vi "Main.vi"() -> (11 "server endpoint URL":string="opc.tcp://10.131.1.22:4840")   [LabVIEW 2018, in "OPC UA.lvlib"]
uses:
  OPC UA.lvlib
  support/Message Queue/Message Cluster.ctl
  <vilib>/Utility/miscctls.llb/LVPoint32TypeDef.ctl
  controls/UI State.ctl
  OPC Module Config.ctl
  Scale Module Folder/Measure Instrument/State Enum.ctl
  OPC Settings.ctl
  Variable Data Cluster.ctl
  <vilib>/OPCUA/controls/NodeId.ctl
  <vilib>/OPCUA/controls/OPC UA StatusCode.ctl
  <vilib>/OPCUA/controls/Subscription ID.ctl
  <vilib>/OPCUA/controls/OPC UA Client Refnum.ctl
  <vilib>/OPCUA/controls/Subscription Data Change.ctl
  <vilib>/OPCUA/controls/Data Type.ctl
  OPC Display Cluster.ctl
  support/Message Queue/Enqueue Message (Single).vi
  <vilib>/Utility/error.llb/Error Cluster From Error Code.vi
  <vilib>/ErrorRing/Error Ring.xnode
  support/Message Queue/Message Queue.lvlib
  support/Support Library.lvlib
  support/Command Log VIs/Command Logging.lvlib
  support/User Event - Stop/User Event - Stop.lvlib
  Scale Module Folder/Measure Instrument/Scale Module Engine.lvlib
  OPC Dialog.vi
panel:
  out "Updating":bool
  in  "Name of Parent Panel":string="Main.vi"
  in  "New Center Coords":T1={"Horizontal"=470, "Vertical"=200}
  in  "Config":variant
  in  "Main UI Message Queue":refnum<queue>
  out "ScanCode":i16
  in  "Settings Button":bool
  in  "Exit":bool
  out "Status":string
  out "Log File path":path
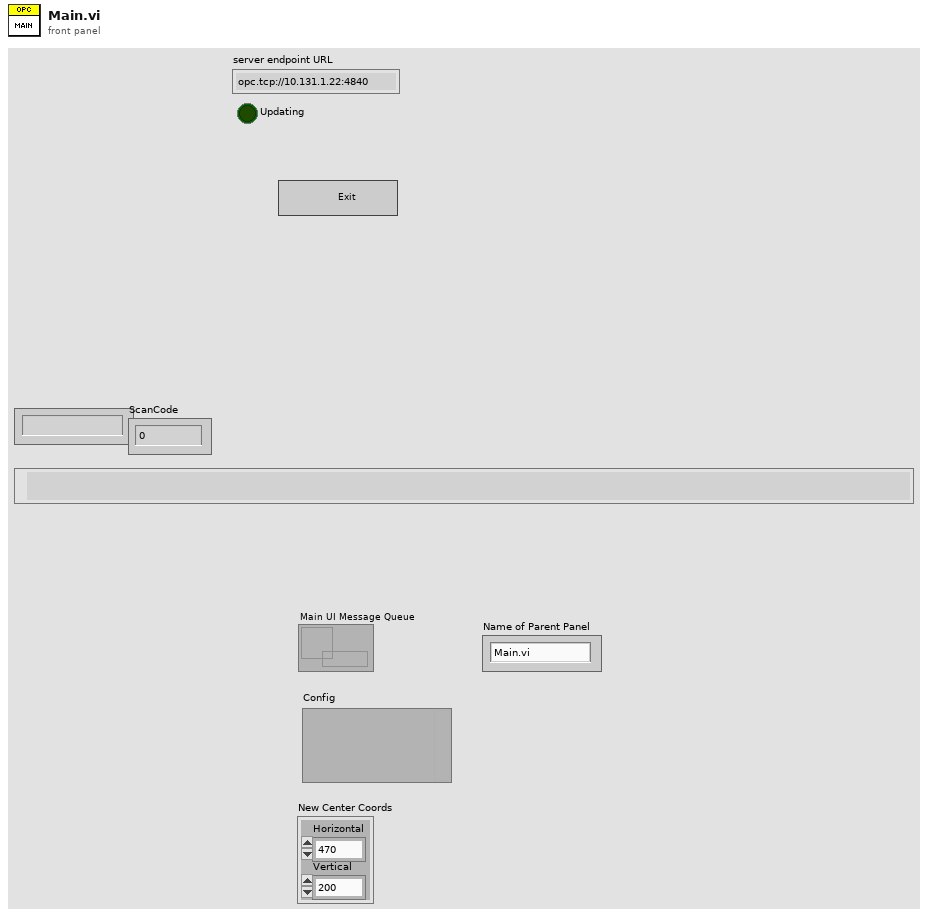
[diagram p1: front panel]
types:
  T1 = typedef "LVPoint32TypeDef.ctl" = cluster{"Horizontal":i32, "Vertical":i32}
  T2 = typedef "UI State.ctl" = enum16{"Idle", "Acquiring and Logging", "Waiting for Exit", "Waiting for Exit (Acq Stopped)", "Waiting for Exit (Log Stopped)", "Waiting for Stop", "Waiting for Stop (Acq Stopped)", "Waiting for Stop (Log Stopped)"}
  T3 = typedef "OPC UA.lvlib/OPC Module Config.ctl" = cluster{"State":T4, "GUID":string, "Drop Coords":T1, "Configuration":T5, "First Iteration":bool, "Data":cluster{"Object Name":string, "Variable Array":T6[]}[], "Process Name":string, "Load Count":i32, "Log Started":bool, "subscription ID out":T9, "OPC UA client refnum out":T10, "Event Registration Refnum":refnum<event-registration>, "Start Time":timestamp, "Current Time":timestamp}
  T4 = typedef "Scale Module.lvlib/Scale Module Engine.lvlib/State Enum.ctl" = enum16{"Measuring", "Idle"}
  T5 = typedef "OPC UA.lvlib/OPC Settings.ctl" = cluster{"Cycle Period":dbl, "server endpoint URL":string, "security policy":cluster{"message mode":enum16{"None", "Sign", "Sign and Encrypt"}, "security":enum16{"Basic256", "Basic128Rsa15"}}, "Trust Any Server":bool}
  T6 = typedef "OPC UA.lvlib/Variable Data Cluster.ctl" = cluster{"node ID":T7, "browse name":string, "status":T8, "timestamp":timestamp, "value ":variant}
  T7 = typedef "NodeId.ctl" = string
  T8 = typedef "OPC UA StatusCode.ctl" = u32
  T9 = typedef "Subscription ID.ctl" = u32
  T10 = typedef "OPC UA Client Refnum.ctl" = refnum<k21>
  T11 = typedef "OPC UA.lvlib/Message Queues.ctl" = cluster{"OPC UI":refnum<queue>, "OPC Engine":refnum<queue>, "OPC Display":refnum<queue>}
  T12 = typedef "OPC UA.lvlib/OPC Display Cluster.ctl" = cluster{"URL":string, "Cycle":i32, "Updating":bool}
  T13 = cluster{"Shift":bool, "Ctrl":bool, "Alt":bool, "Cmd":bool, "Opt":bool}
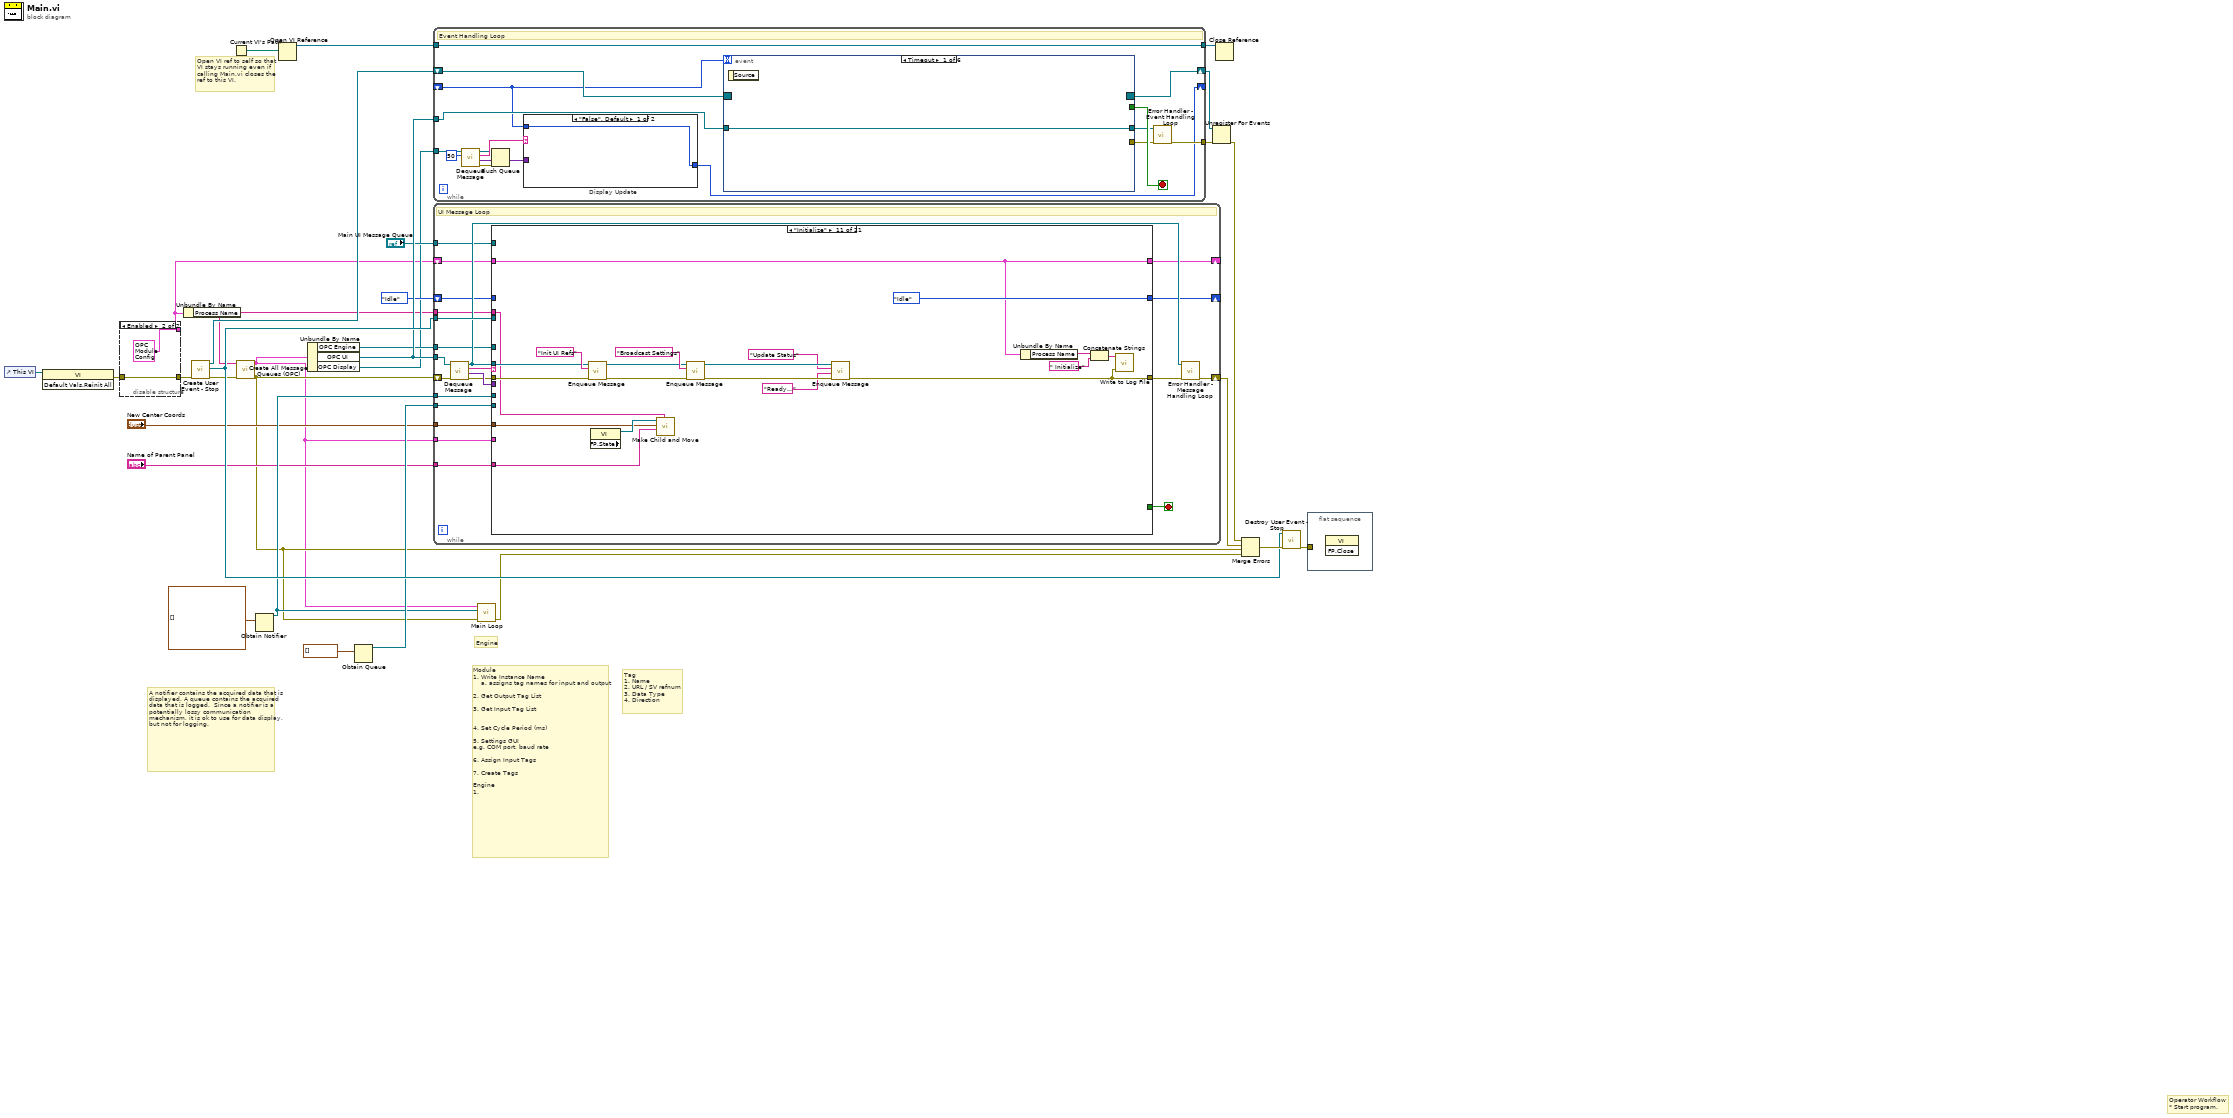
[diagram p0: block diagram]
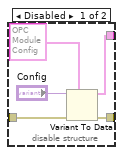
[diagram p2: hidden frame]
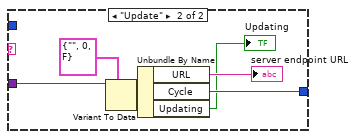
[diagram p3: hidden frame]
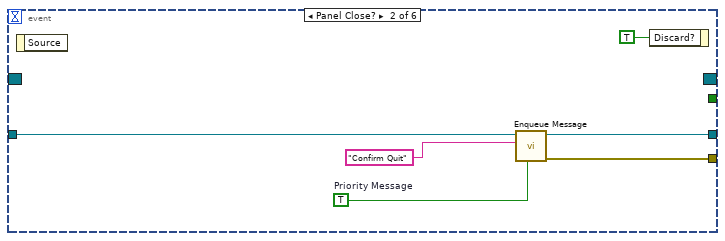
[diagram p4: hidden frame]
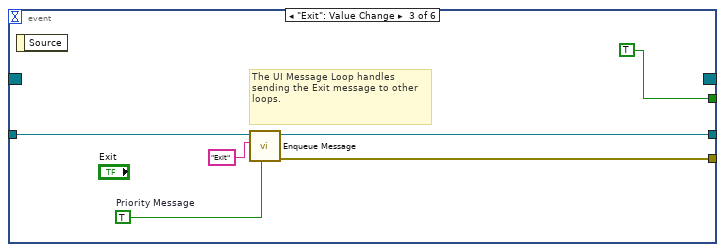
[diagram p5: hidden frame]
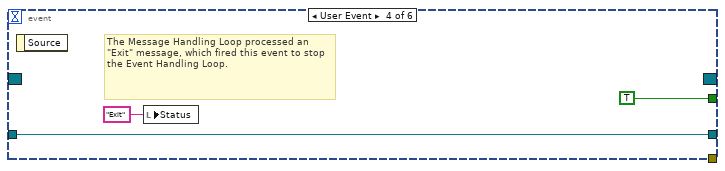
[diagram p6: hidden frame]
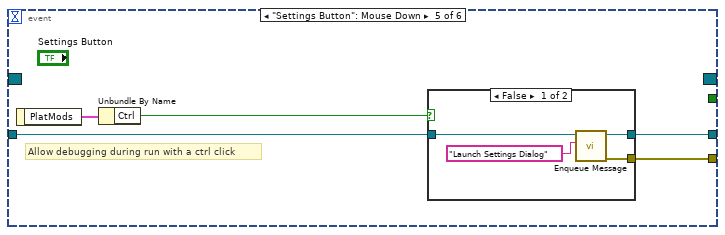
[diagram p7: hidden frame]
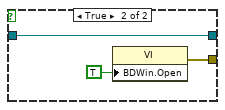
[diagram p8: hidden frame]
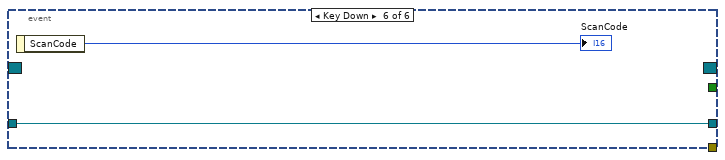
[diagram p9: hidden frame]
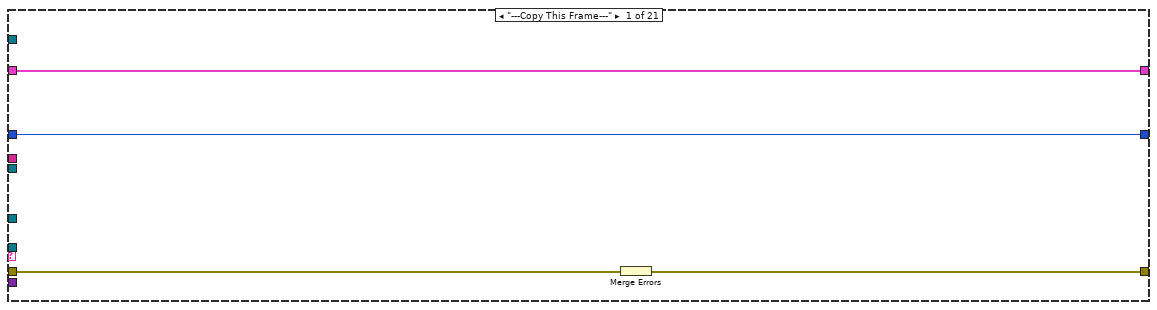
[diagram p10: hidden frame]
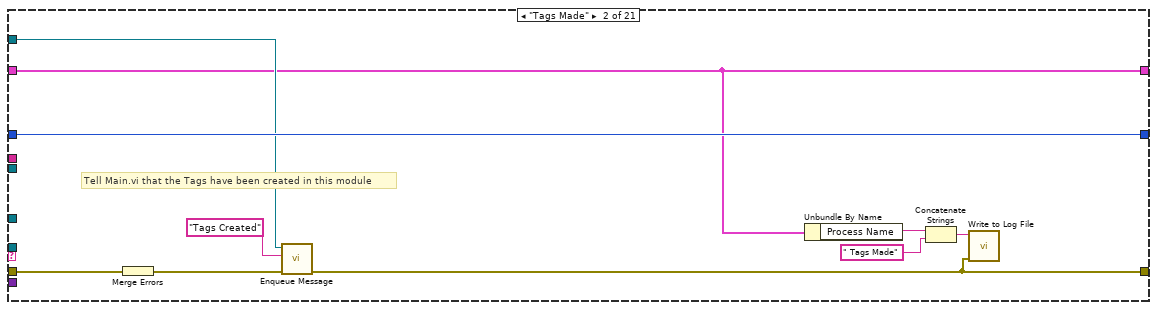
[diagram p11: hidden frame]
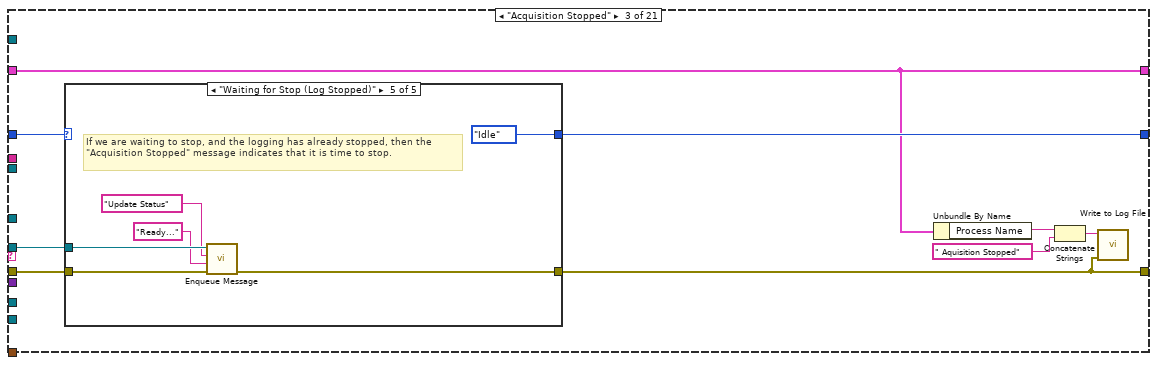
[diagram p12: hidden frame]
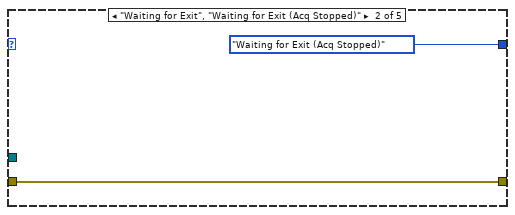
[diagram p14: hidden frame]
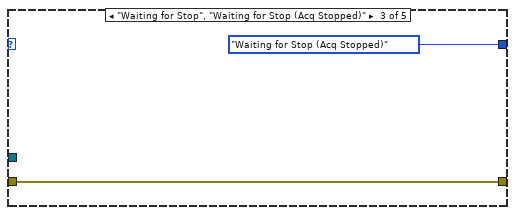
[diagram p15: hidden frame]
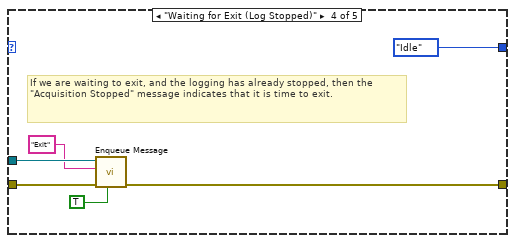
[diagram p16: hidden frame]
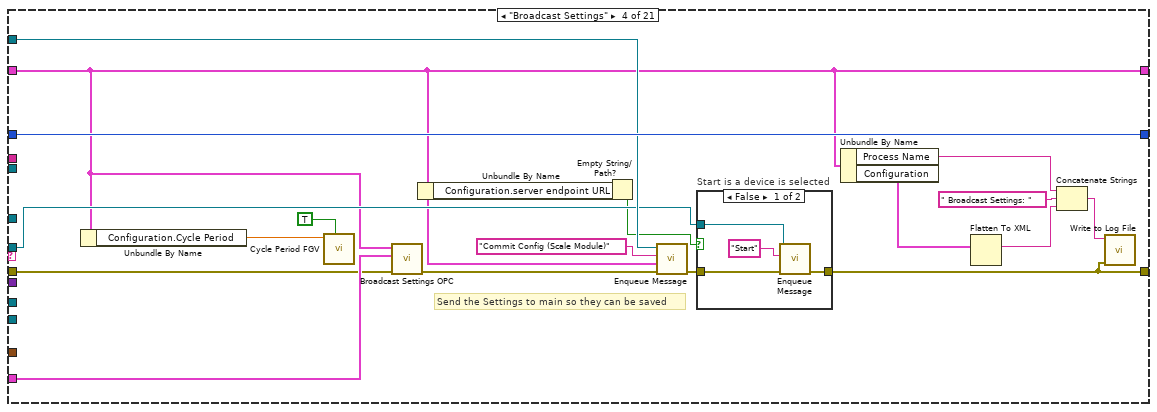
[diagram p17: hidden frame]
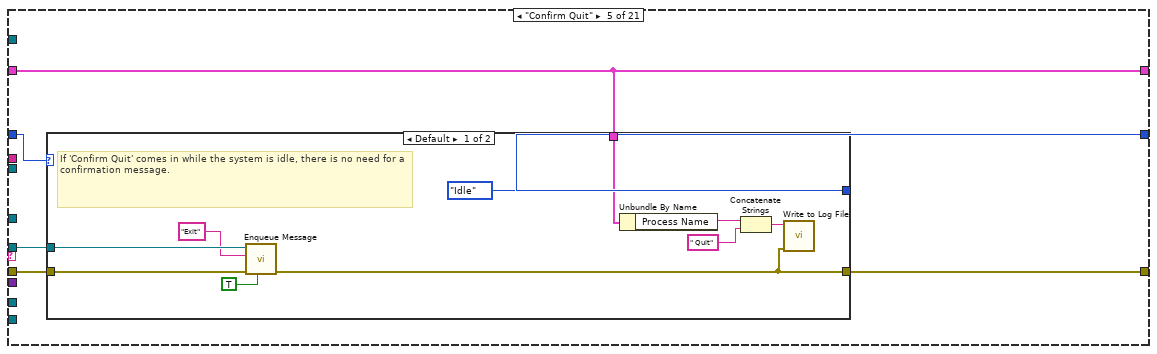
[diagram p19: hidden frame]
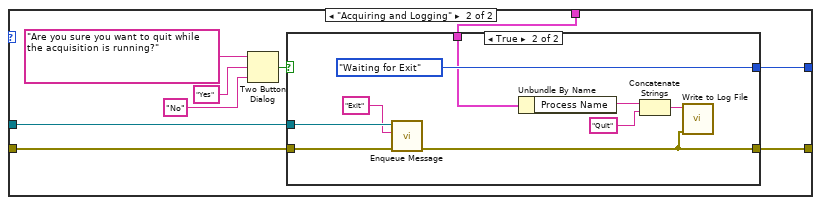
[diagram p20: hidden frame]
diagram:
  # "Open VI ref to self so that\nVI stays running even if\ncalling Main.vi closes the\nref to this VI."
  # "Engine"
  # "Operator Workflow\n* Start program."
  # "Module \n1. Write Instance Name\n    a. assigns tag names for input and output\n\n2. Get Output Tag List\n\n3. Get Input Tag List\n\n\n4. Set Cycle Period (ms)\n\n5. Settings GUI\ne.g. COM port, baud rate\n\n6. Assign Input Tags\n\n7. Create Tags\n\nEngine\n1."
  # "Tag\n1. Name\n2. URL / SV refnum\n3. Data Type\n4. Direction"
  # "A notifier contains the acquired data that is displayed. A queue contains the acquired data that is logged.  Since a notifier is a potentially lossy communication mechanism, it is ok to use for data display, but not for logging."
  n1 = control-ref of="This VI"() -> (w9:refnum<vi>)
  n2 = invoke class="VI" method="Default Vals.Reinit All"(reference=w9) -> (error out=w5:errorcluster)  [unwired: 2 in, 2 out]
  n3 = disable-structure shown="Enabled" {
    disable-tunnel: [w36 w37] -> w13
    disable-tunnel: [w35 T3 {"State"=enum."Idle", "GUID"="", "Drop Coords"={"Horizontal"=0, "Vertical"=0}, "Configuration"={"Cycle Period"=500.0, "server endpoint URL"="opc.tcp://10.131.1.22:4840", "security policy"={"message mode"=enum."Sign", "security"=enum."Basic256"}, "Trust Any Server"=FALSE}, "First Iteration"=FALSE, "Data"=[], "Process Name"="", "Load Count"=0, "Log Started"=FALSE, "subscription ID out"=0, "OPC UA client refnum out"="", "Event Registration Refnum"=refnum, "Start Time"=timestamp(0 s since 1904-01-01), "Current Time"=timestamp(0 s since 1904-01-01)} ("OPC Module Config")] -> w10
    disable-tunnel: w5 -> [w33 w37]
    frame Disabled {
      n4 = Variant To Data(error in=w33, type=T3 {"State"=enum."Idle", "GUID"="", "Drop Coords"={"Horizontal"=0, "Vertical"=0}, "Configuration"={"Cycle Period"=500.0, "server endpoint URL"="opc.tcp://10.131.1.22:4840", "security policy"={"message mode"=enum."Sign", "security"=enum."Basic256"}, "Trust Any Server"=FALSE}, "First Iteration"=FALSE, "Data"=[], "Process Name"="", "Load Count"=0, "Log Started"=FALSE, "subscription ID out"=0, "OPC UA client refnum out"="", "Event Registration Refnum"=refnum, "Start Time"=timestamp(0 s since 1904-01-01), "Current Time"=timestamp(0 s since 1904-01-01)} ("OPC Module Config"), Variant="Config") -> (data=w35:T3, error out=w36:errorcluster)
    }
    frame Enabled {
    }
  }
  n5 = Unbundle By Name(w10) -> ("Process Name"=w4:string)
  n6 = call "Create User Event - Stop.vi"("error in (no error)"=w13) -> ("error out"=w3:errorcluster, "User Event - Stop"=w27:refnum<user-event>, "Stop Event Registration Refnum"=w28:refnum<event-registration>)  [unwired: 8 in]
  n7 = Current VI's Path() -> (path=w14:path)
  n8 = call "Create All Message Queues (OPC).vi"("error in (no error)"=w3, "Process Name"=w4) -> ("error out"=w2:errorcluster, "Message Queues"=w1:T11)  [unwired: 8 in]
  n9 = Obtain Notifier(notification data type=waveform(dbl)[] []) -> (notifier out=w17:refnum<notifier>)  [unwired: 3 in, 2 out]
  n10 = Open VI Reference(vi path=w14) -> (vi reference=w15:refnum<vi>)  [unwired: 5 in, 1 out]
  n11 = Unbundle By Name(w1) -> ("OPC Engine"=w20:refnum<queue>, "OPC UI"=w24:refnum<queue>, "OPC Display"=w11:refnum<queue>)
  n12 = Obtain Queue(element data type=waveform(dbl)[] []) -> (queue out=w19:refnum<queue>)  [unwired: 4 in, 2 out]
  n13 = while {
    tunnel: w24 -> [w55]
    tunnel: w27 -> [w59]
    shift-right: [w51] -> w31
    shift-left: w2 -> [w58]
    shift-right: [w42] -> _
    shift-left: w10 -> [w44]
    tunnel: w17 -> [w54]
    tunnel: w19 -> [w53]
    shift-right: [w48] -> _
    shift-left: UI_State."Idle" ("UI State") -> [w49]
    tunnel: w20 -> [w47]
    tunnel: w1 -> [w46]
    tunnel: "Main UI Message Queue" -> [w43]
    tunnel: w4 -> [w41]
    tunnel: "New Center Coords" -> [w40]
    tunnel: "Name of Parent Panel" -> [w39]
    stop <- w60 stop-if-true
    # "UI Message Loop"
    n14 = call "Dequeue Message.vi"("error in (no error)"=w58, "Message Queue"=w55) -> ("error out"=w45:errorcluster, "Message Data"=w56:variant, "Message"=w57:string, "dup Message Queue"=w50:refnum<queue>)  [unwired: 6 in]
    n15 = case "Message Cases" shown="\"Initialize\"" w57 {
      selector: w57 -> [_ _ _ _ _ _ _ _ _ _ _ _ _ _ _ _ _ _ _ _ w395]
      tunnel: w50 -> [_ _ w80 w115 w130 _ w180 w194 w216 _ w255 w272 w288 w311 w319 w337 _ _ w384 _ _]
      tunnel: w45 -> [w64 w74 w81 w103 w129 w164 w175 w198 w215 w241 w251 w264 w289 w312 w318 w336 w343 w360 w379 w393 _]
      tunnel: [w63 w65 w76 w110 w128 w165 w170 w185 w200 w241 w243 w268 w284 w310 w317 w332 w348 w355 w371 w394 w397] -> w52
      tunnel: [_ _ _ _ _ _ _ _ TRUE _ _ _ _ _ _ _ _ _ _ _ _] -> w60
      tunnel: w56 -> [_ _ _ _ _ w167 _ w197 w205 _ _ _ _ _ _ _ _ _ _ w392 _]
      tunnel: w59 -> [_ _ _ _ _ _ _ _ w226 _ _ _ _ _ _ _ _ _ _ _ _]
      tunnel: w44 -> [w61 w66 w75 w109 w126 w162 w169 w184 w199 w238 w242 w267 w283 w316 w323 w331 w341 w354 w370 w387 w396]
      tunnel: w54 -> [_ _ _ _ _ _ _ _ w224 _ _ _ _ _ _ _ _ _ _ _ _]
      tunnel: w53 -> [_ _ _ _ _ _ _ _ w220 _ _ _ _ _ _ _ _ _ _ _ _]
      tunnel: w49 -> [w62 w73 w83 w120 w131 w163 w176 w189 w213 _ _ w276 w291 w315 w322 _ _ _ w380 w388 w401]
      tunnel: [w62 w73 w82 w120 w127 w163 w177 w189 w212 UI_State."Idle" ("UI State") UI_State."Idle" ("UI State") w276 w290 w315 w322 UI_State."Acquiring and Logging" ("UI State") UI_State."Acquiring and Logging" ("UI State") UI_State."Acquiring and Logging" ("UI State") w381 w388 w401] -> w48
      tunnel: w47 -> [_ _ _ _ _ _ _ _ w219 _ _ _ _ _ _ _ w346 w363 w378 _ _]
      tunnel: w46 -> [_ _ _ w104 _ _ _ _ _ _ _ _ _ _ _ _ _ _ _ _ _]
      tunnel: w43 -> [_ w70 _ w116 _ _ _ _ w204 _ _ w273 _ _ _ _ _ _ _ _ _]
      tunnel: [w61 w66 w75 w109 w126 w162 w169 w184 w199 w238 w242 w262 w283 w316 w323 w331 w341 w354 w370 w387 w396] -> w42
      tunnel: w41 -> [_ _ _ _ _ _ _ _ _ _ w249 _ _ _ _ _ _ _ _ _ _]
      tunnel: w40 -> [_ _ _ _ _ _ _ _ _ _ w248 _ _ _ _ _ _ _ _ _ _]
      tunnel: w39 -> [_ _ _ _ _ _ _ _ _ _ w247 _ _ _ _ _ _ _ _ _ _]
      frame "---Copy This Frame---" {
        # "Duplicate this frame when creating new messages.  Change this comment in the duplicated frame to describe this message."
        n16 = Merge Errors(w64) -> (w63:errorcluster)
      }
      frame "Tags Made" {
        # "Tell Main.vi that the Tags have been created in this module"
        # "Duplicate this frame when creating new messages.  Change this comment in the duplicated frame to describe this message."
        n17 = Merge Errors(w74) -> (w71:errorcluster)
        n18 = call-poly "Enqueue Message.vi"("error in (no error)"=w71, "Message"="Tags Created", "Message Queue"=w70) -> ("error out"=w65:errorcluster)  [unwired: 7 in, 1 out]
        n19 = Unbundle By Name(w66) -> ("Process Name"=w69:string)
        n20 = Concatenate Strings(w69, " Tags Made" ("text")) -> (w67:string)
        n21 = call "Write to Log File.vi"("error in"=w65, "text"=w67) -> ()  [unwired: 9 in, 1 out]
      }
      frame "Acquisition Stopped" {
        # "Logic for determining what action to take when the acquisition has stopped."
        n22 = case shown="\"Waiting for Stop (Log Stopped)\"" w83 {
          selector: w83 -> [w85 _ _ _ _]
          tunnel: [w85 UI_State."Waiting for Exit (Acq Stopped)" ("UI State") UI_State."Waiting for Stop (Acq Stopped)" ("UI State") UI_State."Idle" ("UI State") UI_State."Idle" ("UI State")] -> w82
          tunnel: w81 -> [w84 w86 w88 w94 w100]
          tunnel: [w84 w86 w88 w93 w99] -> w76
          tunnel: w80 -> [_ _ _ w92 w98]
          frame Default {
          }
          frame "Waiting for Exit", "Waiting for Exit (Acq Stopped)" {
          }
          frame "Waiting for Stop", "Waiting for Stop (Acq Stopped)" {
          }
          frame "Waiting for Exit (Log Stopped)" {
            # "If we are waiting to exit, and the logging has already stopped, then the \"Acquisition Stopped\" message indicates that it is time to exit."
            n23 = call-poly "Enqueue Message.vi"("Priority Message? (F)"=TRUE, "error in (no error)"=w94, "Message"="Exit", "Message Queue"=w92) -> ("error out"=w93:errorcluster)  [unwired: 6 in, 1 out]
          }
          frame "Waiting for Stop (Log Stopped)" {
            # "If we are waiting to stop, and the logging has already stopped, then the \"Acquisition Stopped\" message indicates that it is time to stop."
            n24 = call-poly "Enqueue Message.vi"("error in (no error)"=w100, "Message Data"="Ready..." ("Message"), "Message"="Update Status", "Message Queue"=w98) -> ("error out"=w99:errorcluster)  [unwired: 6 in, 1 out]
          }
        }
        n25 = Unbundle By Name(w75) -> ("Process Name"=w79:string)
        n26 = Concatenate Strings(w79, " Aquisition Stopped" ("text")) -> (w77:string)
        n27 = call "Write to Log File.vi"("error in"=w76, "text"=w77) -> ()  [unwired: 9 in, 1 out]
      }
      frame "Broadcast Settings" {
        # "Send the Settings to main so they can be saved"
        # "Send the 'Update Settings' message to the Logging and Acquisition message loops."
        n28 = Unbundle By Name(w109) -> ("Configuration.Cycle Period"=w118:dbl)
        n29 = call "Cycle Period FGV.vi"("Write"=TRUE, "Cycle Period In (ms)"=w118) -> ()  [unwired: 8 in, 2 out]
        n30 = call "Broadcast Settings OPC.vi"("error in (no error)"=w103, "Message Queues"=w104, "OPC Module Config"=w109) -> ("error out"=w102:errorcluster)  [unwired: 8 in]
        n31 = Unbundle By Name(w109) -> ("Configuration.server endpoint URL"=w106:string)
        n32 = Empty String/Path?(string/path=w106) -> (empty?=w105:bool)
        n33 = call-poly "Enqueue Message.vi"("error in (no error)"=w102, "Message Data"=w109, "Message"="Commit Config (Scale Module)", "Message Queue"=w116) -> ("error out"=w114:errorcluster)  [unwired: 6 in, 1 out]
        n34 = case "Start is a device is selected" shown="False" w105 {
          tunnel: w115 -> [w123 _]
          tunnel: w114 -> [w122 w125]
          tunnel: [w121 w125] -> w110
          frame False {
            n35 = call-poly "Enqueue Message.vi"("error in (no error)"=w122, "Message"="Start", "Message Queue"=w123) -> ("error out"=w121:errorcluster)  [unwired: 7 in, 1 out]
          }
          frame True {
          }
        }
        n36 = Unbundle By Name(w109) -> ("Process Name"=w113:string, "Configuration"=w108:T5)
        n37 = Flatten To XML(anything=w108) -> (xml string=w107:string)
        n38 = Concatenate Strings(w113, " Broadcast Settings: " ("text"), w107) -> (w111:string)
        n39 = call "Write to Log File.vi"("error in"=w110, "text"=w111) -> ()  [unwired: 9 in, 1 out]
      }
      frame "Confirm Quit" {
        # "Confirm Quit - Message that can confirm whether or not the user wants to exit the application."
        n40 = case shown="Default" w131 {
          tunnel: w130 -> [w140 w147]
          tunnel: w129 -> [w139 w145]
          tunnel: [w133 w144] -> w128
          tunnel: [UI_State."Idle" ("UI State") w143] -> w127
          tunnel: w126 -> [w132 w142]
          frame Default {
            # "If 'Confirm Quit' comes in while the system is idle, there is no need for a confirmation message."
            n41 = call-poly "Enqueue Message.vi"("Priority Message? (F)"=TRUE, "error in (no error)"=w139, "Message"="Exit", "Message Queue"=w140) -> ("error out"=w133:errorcluster)  [unwired: 6 in, 1 out]
            n42 = Unbundle By Name(w132) -> ("Process Name"=w136:string)
            n43 = Concatenate Strings(w136, " Quit" ("text")) -> (w134:string)
            n44 = call "Write to Log File.vi"("error in"=w133, "text"=w134) -> ()  [unwired: 9 in, 1 out]
          }
          frame "Acquiring and Logging" {
            n45 = Two Button Dialog(message="Are you sure you want to quit while the acquisition is running?" ("Confirm Quit Message"), 1:"No" ("No"), 2:"Yes" ("Yes")) -> (T button?=w146:bool)
            n46 = case shown="True" w146 {
              tunnel: w147 -> [_ w161]
              tunnel: w145 -> [w151 w160]
              tunnel: [w151 w154] -> w144
              tunnel: [UI_State."Acquiring and Logging" ("UI State") UI_State."Waiting for Exit" ("UI State")] -> w143
              tunnel: w142 -> [_ w153]
              frame False {
                # "User did not want to quit."
              }
              frame True {
                n47 = call-poly "Enqueue Message.vi"("error in (no error)"=w160, "Message"="Exit", "Message Queue"=w161) -> ("error out"=w154:errorcluster)  [unwired: 7 in, 1 out]
                n48 = Unbundle By Name(w153) -> ("Process Name"=w157:string)
                n49 = Concatenate Strings(w157, "Quit" ("text")) -> (w155:string)
                n50 = call "Write to Log File.vi"("error in"=w154, "text"=w155) -> ()  [unwired: 9 in, 1 out]
              }
            }
          }
        }
      }
      frame "Display Log File Path" {
        n51 = Variant To Data(error in=w164, type=path "", Variant=w167) -> (data=→"Log File path":path, error out=w165:errorcluster)
      }
      frame "E-Stop" {
        # "E-Stop has no effect on the scale"
        # "Message Acquisition and Logging loops to stop"
        # "Stop the pumps."
        n52 = call-poly "Enqueue Message.vi"("error in (no error)"=w175, "Message Data"="Ready..." ("Ready..."), "Message"="Update Status", "Message Queue"=w180) -> ("error out"=w174:errorcluster)  [unwired: 6 in, 1 out]
        n53 = case shown="\"Waiting for Exit\"" w176 {
          selector: w176 -> [_ w182]
          tunnel: [UI_State."Waiting for Stop" ("UI State") w182] -> w177
          frame Default {
          }
          frame "Waiting for Exit" {
          }
        }
        n54 = Merge Errors(w174) -> (w170:errorcluster)
        n55 = Unbundle By Name(w169) -> ("Process Name"=w173:string)
        n56 = Concatenate Strings(w173, " E-STOP" ("text")) -> (w171:string)
        n57 = call "Write to Log File.vi"("error in"=w170, "text"=w171) -> ()  [unwired: 9 in, 1 out]
      }
      frame "Error" {
        # "Error - Check the error message data and respond accordingly. This message is sent by the \"Error Handler\" VIs at the end of each loop in this application."
        n58 = Variant To Data(error in=w198, type=errorcluster {"status"=FALSE, "code"=0, "source"=""} ("error out"), Variant=w197) -> (data=w195:errorcluster, error out=w191:errorcluster)
        n59 = call <vilib>:"General Error Handler.vi"("error in (no error)"=w195) -> ("message"=w183:string)  [unwired: 10 in, 4 out]
        n60 = call-poly "Enqueue Message.vi"("Priority Message? (F)"=TRUE, "Message"="Exit", "Message Queue"=w194) -> ("error out"=w190:errorcluster)  [unwired: 7 in, 1 out]
        n61 = Merge Errors(w190, w191) -> (w185:errorcluster)
        n62 = Unbundle By Name(w184) -> ("Process Name"=w188:string)
        n63 = Concatenate Strings(w188, " Error: " ("text"), w183) -> (w186:string)
        n64 = call "Write to Log File.vi"("error in"=w185, "text"=w186) -> ()  [unwired: 9 in, 1 out]
      }
      frame "Exit" {
        w208 = TRUE  # Delete Module?
        # "Don't check the error outs. The acquisition and logging queues may have already been released."
        # "Close references owned by the Main VI."
        # "Stop the VI"
        # "Exit - Fire the User Event to stop the Event Handling Loop.  Also send Exit messages to the Acquisition and Logging loops."
        n65 = call "Fire User Event - Stop.vi"("User Event - Stop"=w226) -> ("error out"=w225:errorcluster)  [unwired: 10 in]
        n66 = Build Array(w219) -> (w218:refnum<queue>[])
        n67 = for {
          tunnel: w218 -> [w235] mode=indexing
          n68 = call-poly "Enqueue Message.vi"("Message"="Stop", "Message Queue"=w235) -> ("dup Message Queue"=w236:refnum<queue>)  [unwired: 8 in, 1 out]
          n69 = call-poly "Enqueue Message.vi"("Message"="Exit", "Message Queue"=w236) -> ()  [unwired: 8 in, 2 out]
        }
        n70 = Variant To Data(type=w208, Variant=w205) -> (data=w207:bool, error out=w209:errorcluster)  [unwired: 1 in]
        n71 = call-poly "Enqueue Message.vi"("error in (no error)"=w215, "Message Data"="Ready..." ("Ready..."), "Message"="Update Status", "Message Queue"=w216) -> ("error out"=w214:errorcluster, "dup Message Queue"=w211:refnum<queue>)  [unwired: 6 in]
        n72 = Select(t=w208, s=w209, f=w207) -> (s? t:f=w206:bool)
        n73 = case "Don't enqueue Delete Module if opening campaign because it\nwill already have been deleted and new config loaded and we create\na race condition." shown="True" w206 {
          tunnel: w204 -> [_ w230]
          tunnel: w199 -> [_ w229]
          frame False {
          }
          frame True {
            n74 = Unbundle By Name(w229) -> ("GUID"=w228:string)
            n75 = call-poly "Enqueue Message.vi"("Message Data"=w228, "Message"="Delete Module", "Message Queue"=w230) -> ()  [unwired: 7 in, 2 out]
          }
        }
        n76 = Release Queue(queue=w211, error in (no error)=w214) -> (error out=w223:errorcluster)  [unwired: 1 in, 2 out]
        n77 = Release Notifier(notifier=w224, error in (no error)=w223) -> (error out=w222:errorcluster)  [unwired: 1 in, 2 out]
        n78 = Release Queue(queue=w220, error in (no error)=w222) -> (error out=w221:errorcluster)  [unwired: 1 in, 2 out]
        n79 = Merge Errors(w225, w221) -> (w200:errorcluster)
        n80 = case shown="Default" w213 {
          selector: w213 -> [_ w233]
          tunnel: [UI_State."Waiting for Stop" ("UI State") w233] -> w212
          frame Default {
          }
          frame "Waiting for Exit" {
          }
        }
        n81 = Unbundle By Name(w199) -> ("Process Name"=w203:string)
        n82 = Concatenate Strings(w203, " Exit" ("text")) -> (w201:string)
        n83 = call "Write to Log File.vi"("error in"=w200, "text"=w201) -> ()  [unwired: 9 in, 1 out]
      }
      frame "Init UI Refs" {
        # "Init UI Refs - Store control references for UI controls.  Also enable/disable controls appropriately."
        n84 = property class="VI"("Front Panel.Closeable"=TRUE ("Front Panel Window:Closeable")) -> ()  [unwired: 2 in, 2 out]
      }
      frame "Initialize" {
        # "Initialize - Get configuration settings, then message the UI to initialize, and broadcast the settings to the other message loops."
        n85 = call-poly "Enqueue Message.vi"("error in (no error)"=w251, "Message"="Init UI Refs", "Message Queue"=w255) -> ("error out"=w253:errorcluster, "dup Message Queue"=w254:refnum<queue>)  [unwired: 7 in]
        n86 = property class="VI" props=["FP.State"]() -> (reference out=w250:refnum<vi>)  [unwired: 2 in, 2 out]
        n87 = call "Make Child and Move.vi"("Process Name"=w249, "Name of Parent Panel"=w247, "New Center Coords"=w248, "VI in"=w250) -> ()  [unwired: 8 in]
        n88 = call-poly "Enqueue Message.vi"("error in (no error)"=w253, "Message"="Broadcast Settings", "Message Queue"=w254) -> ("error out"=w261:errorcluster, "dup Message Queue"=w260:refnum<queue>)  [unwired: 7 in]
        n89 = call-poly "Enqueue Message.vi"("error in (no error)"=w261, "Message Data"="Ready..." ("Ready..."), "Message"="Update Status", "Message Queue"=w260) -> ("error out"=w243:errorcluster)  [unwired: 6 in, 1 out]
        n90 = Unbundle By Name(w242) -> ("Process Name"=w246:string)
        n91 = Concatenate Strings(w246, " Initialize" ("text")) -> (w244:string)
        n92 = call "Write to Log File.vi"("error in"=w243, "text"=w244) -> ()  [unwired: 9 in, 1 out]
      }
      frame "Launch Settings Dialog" {
        # "Launch the Settings Dialog when the user clicks the 'Settings' button."
        n93 = Unbundle By Name(w267) -> ("Load Count"=w274:i32)
        n94 = Increment(x=w274) -> (x+1=w275:i32)
        n95 = Bundle By Name(cluster=w267, "Load Count"=w275) -> (w263:T3)
        n96 = call-by-ref "?"("error in (no error)"=w264, "OPC Module Config In"=w263) -> ("error out"=w265:errorcluster, "Cancelled?"=w266:bool, "OPC Module Config Out"=w262:T3)  [unwired: 8 in, 3 out]
        n97 = case shown="False" w266 {
          tunnel: w265 -> [w279 w282]
          tunnel: [w278 w282] -> w268
          tunnel: w273 -> [_ _]
          tunnel: w272 -> [w281 _]
          tunnel: w262 -> [w277 _]
          frame False {
            n98 = call-poly "Enqueue Message.vi"("error in (no error)"=w279, "Message Data"=w277, "Message"="Broadcast Settings", "Message Queue"=w281) -> ("error out"=w278:errorcluster)  [unwired: 6 in, 1 out]
          }
          frame True {
          }
        }
        n99 = Unbundle By Name(w262) -> ("Process Name"=w271:string)
        n100 = Concatenate Strings(w271, " Setting Dialog Launched" ("text")) -> (w269:string)
        n101 = call "Write to Log File.vi"("error in"=w268, "text"=w269) -> ()  [unwired: 9 in, 1 out]
      }
      frame "Logging Stopped" {
        # "Logic for determining what action to take when the logging has stopped."
        n102 = case shown="\"Waiting for Exit (Acq Stopped)\"" w291 {
          selector: w291 -> [w293 _ _ _ _]
          tunnel: [w293 UI_State."Waiting for Exit (Log Stopped)" ("UI State") UI_State."Waiting for Stop (Log Stopped)" ("UI State") UI_State."Idle" ("UI State") UI_State."Idle" ("UI State")] -> w290
          tunnel: w289 -> [w292 w294 w296 w302 w308]
          tunnel: [w292 w294 w296 w301 w307] -> w284
          tunnel: w288 -> [_ _ _ w300 w306]
          frame Default {
          }
          frame "Waiting for Exit", "Waiting for Exit (Log Stopped)" {
          }
          frame "Waiting for Stop", "Waiting for Stop (Log Stopped)" {
          }
          frame "Waiting for Exit (Acq Stopped)" {
            # "If we are waiting to exit, and the acquisition has already stopped, then the \"Logging Stopped\" message indicates that it is time to exit."
            n103 = call-poly "Enqueue Message.vi"("Priority Message? (F)"=TRUE, "error in (no error)"=w302, "Message"="Exit", "Message Queue"=w300) -> ("error out"=w301:errorcluster)  [unwired: 6 in, 1 out]
          }
          frame "Waiting for Stop (Acq Stopped)" {
            # "If we are waiting to stop, and the acquisition has already stopped, then the \"Logging Stopped\" message indicates that it is time to stop."
            n104 = call-poly "Enqueue Message.vi"("error in (no error)"=w308, "Message Data"="Ready..." ("Message"), "Message"="Update Status", "Message Queue"=w306) -> ("error out"=w307:errorcluster)  [unwired: 6 in, 1 out]
          }
        }
        n105 = Unbundle By Name(w283) -> ("Process Name"=w287:string)
        n106 = Concatenate Strings(w287, " Logging Stopped" ("text")) -> (w285:string)
        n107 = call "Write to Log File.vi"("error in"=w284, "text"=w285) -> ()  [unwired: 9 in, 1 out]
      }
      frame "Send to Sequencer" {
        n108 = local read "Status"() -> (w313:string)
        n109 = call-poly "Enqueue Message.vi"("error in (no error)"=w312, "Message Data"=w313, "Message"="Sent to Sequence", "Message Queue"=w311) -> ("error out"=w310:errorcluster)  [unwired: 6 in, 1 out]
      }
      frame "Sent to Sequence" {
        n110 = local read "Status"() -> (w320:string)
        n111 = flat-sequence {
          tunnel: w318 -> [w328]
          tunnel: w319 -> [w326]
          tunnel: [w327] -> w321
          tunnel: w320 -> [w324]
          tunnel: [w330] -> w317
          tunnel: w321 -> [w330]
          frame #0 {
            n112 = call-poly "Enqueue Message.vi"("error in (no error)"=w328, "Message Data"=w324, "Message"="Sent to Sequence", "Message Queue"=w326) -> ("error out"=w327:errorcluster)  [unwired: 6 in, 1 out]
          }
          frame #1 {
            n113 = Wait (ms)(milliseconds to wait=u32 50) -> ()  [unwired: 1 out]
          }
        }
      }
      frame "Start" {
        # "Message Acquisition and Logging loops to start"
        # "Start - Enable/Disable buttons appropriately for an acquisition that has started, and update status display."
        n114 = call-poly "Enqueue Message.vi"("error in (no error)"=w336, "Message"="Start Loops", "Message Queue"=w337) -> ("error out"=w338:errorcluster)  [unwired: 7 in, 1 out]
        n115 = Merge Errors(w338) -> (w332:errorcluster)
        n116 = Unbundle By Name(w331) -> ("Process Name"=w335:string)
        n117 = Concatenate Strings(w335, " Start" ("text")) -> (w333:string)
        n118 = call "Write to Log File.vi"("error in"=w332, "text"=w333) -> ()  [unwired: 9 in, 1 out]
      }
      frame "Start Loops" {
        # "I'm not sure what we would have multiple Process names in a module for but i'll leave it for now."
        # "Message Acquisition and Logging loops to start"
        # "Start - Enable/Disable buttons appropriately for an acquisition that has started, and update status display."
        n119 = Build Array(w346) -> (w344:refnum<queue>[])
        n120 = Unbundle By Name(w341) -> ("Process Name"=w342:string)
        n121 = property class="VI"("Front Panel.Title"=w342) -> ()  [unwired: 2 in, 2 out]
        n122 = for {
          tunnel: w343 -> [w352]
          tunnel: [w351] -> w345 mode=indexing
          tunnel: w344 -> [w350] mode=indexing
          tunnel: w342 -> [w349]
          n123 = call-poly "Enqueue Message.vi"("error in (no error)"=w352, "Message Data"=w349, "Message"="Start", "Message Queue"=w350) -> ("error out"=w351:errorcluster)  [unwired: 6 in, 1 out]
        }
        n124 = Merge Errors(w345) -> (w348:errorcluster)
      }
      frame "Start Log" {
        # "I'm not sure what we would have multiple Process names in a module for but i'll leave it for now."
        # "Message Acquisition and Logging loops to start"
        # "Start - Enable/Disable buttons appropriately for an acquisition that has started, and update status display."
        n125 = Build Array(w363) -> (w361:refnum<queue>[])
        n126 = Unbundle By Name(w354) -> ("Process Name"=w359:string)
        n127 = property class="VI"("Front Panel.Title"=w359) -> ()  [unwired: 2 in, 2 out]
        n128 = for {
          tunnel: w360 -> [w368]
          tunnel: [w367] -> w362 mode=indexing
          tunnel: w361 -> [w366] mode=indexing
          tunnel: w359 -> [w365]
          n129 = call-poly "Enqueue Message.vi"("error in (no error)"=w368, "Message Data"=w365, "Message"="Start Log", "Message Queue"=w366) -> ("error out"=w367:errorcluster)  [unwired: 6 in, 1 out]
        }
        n130 = Merge Errors(w362) -> (w355:errorcluster)
        n131 = Unbundle By Name(w354) -> ("Process Name"=w358:string)
        n132 = Concatenate Strings(w358, " Start Log" ("text")) -> (w356:string)
        n133 = call "Write to Log File.vi"("error in"=w355, "text"=w356) -> ()  [unwired: 9 in, 1 out]
      }
      frame "Stop" {
        # "Stop - Enable/Disable buttons appropriately for an acquisition that has stopped, and update status display."
        n134 = call-poly "Enqueue Message.vi"("error in (no error)"=w379, "Message Data"="Ready..." ("Ready..."), "Message"="Update Status", "Message Queue"=w384) -> ("error out"=w377:errorcluster)  [unwired: 6 in, 1 out]
        n135 = call-poly "Enqueue Message.vi"("error in (no error)"=w377, "Message"="Stop", "Message Queue"=w378) -> ("error out"=w375:errorcluster)  [unwired: 7 in, 1 out]
        n136 = case shown="Default" w380 {
          selector: w380 -> [_ w386]
          tunnel: [UI_State."Waiting for Stop" ("UI State") w386] -> w381
          frame Default {
          }
          frame "Waiting for Exit" {
          }
        }
        n137 = Merge Errors(w375) -> (w371:errorcluster)
        n138 = Unbundle By Name(w370) -> ("Process Name"=w374:string)
        n139 = Concatenate Strings(w374, " Stop" ("text")) -> (w372:string)
        n140 = call "Write to Log File.vi"("error in"=w371, "text"=w372) -> ()  [unwired: 9 in, 1 out]
      }
      frame "Update Status" {
        # "Update Display - Convert the message data to a string to display in the Status indicator."
        n141 = Variant To Data(error in=w393, type="", Variant=w392) -> (data=→"Status":string, error out=w390:errorcluster)
        n142 = Merge Errors(w390) -> (w394:errorcluster)
      }
      frame Default {
        # "'Default' case only runs if there is a message that isn't defined in any of the other cases.  Output a programming error."
        n143 = xnode "Error Ring"("parameter 0"=w395) -> ("error out"=w397:errorcluster)
        n144 = Unbundle By Name(w396) -> ("Process Name"=w400:string)
        n145 = Concatenate Strings(w400, "Invalid Message Recieved" ("text"), w395) -> (w398:string)
        n146 = call "Write to Log File.vi"("error in"=w397, "text"=w398) -> ()  [unwired: 9 in, 1 out]
      }
    }
    n147 = call "Error Handler - Message Handling Loop.vi"("error in (no error)"=w52, "Message Queue"=w50) -> ("dup error in"=w51:errorcluster)  [unwired: 8 in, 1 out]
  }
  n148 = while {
    tunnel: w24 -> [w418]
    tunnel: [w420] -> w30
    shift-right: [w419] -> w25
    shift-left: w28 -> [w424]
    tunnel: [w417] -> w16
    tunnel: w15 -> [w417]
    tunnel: w11 -> [w416]
    shift-right: [w409] -> _
    shift-left: _ -> [w410]
    stop <- w423 stop-if-true
    # "Event Handling Loop"
    n149 = call "Dequeue Message.vi"("timeout in ms (-1)"=50, "Message Queue"=w416) -> ("error out"=w411:errorcluster, "Message Data"=w414:variant, "Message"=w415:string, "dup Message Queue"=w412:refnum<queue>)  [unwired: 6 in]
    n150 = Flush Queue(queue=w412, error in (no error)=w411) -> ()  [unwired: 3 out]
    n151 = case "Display Update" shown="\"False\", Default" w415 {
      tunnel: w414 -> [_ w431]
      tunnel: w410 -> [w425 _]
      tunnel: [w425 w428] -> w409
      frame "False", Default {
      }
      frame "Update" {
        n152 = Variant To Data(type=T12 {"URL"="", "Cycle"=0, "Updating"=FALSE} ("OPC Display Cluster"), Variant=w431) -> (data=w430:T12)  [unwired: 1 in, 1 out]
        n153 = Unbundle By Name(w430) -> ("URL"=→"server endpoint URL":string, "Cycle"=w428:i32, "Updating"=→"Updating":bool)
      }
    }
    n154 = event shown="[0] Timeout" {
      selector: w424 -> [_ _ _ _ _ _]
      dyn-events: [_ _ _ _ _ _] -> w419
      timeout: w410 -> [_ _ _ _ _ _]
      tunnel: [_ _ TRUE ("Discard?") TRUE ("Discard?") _ _] -> w423
      tunnel: w418 -> [w432 w435 w439 w445 w450 w460]
      tunnel: [_ w433 w444 _ w452 _] -> w421
      tunnel: [w432 w434 w442 w445 w451 w460] -> w422
      event Timeout {
        n155 = event-data() -> ()  [unwired: 1 in, 1 out]
      }
      event Panel Close? {
        w436 = TRUE  # Priority Message
        n156 = event-data() -> ()  [unwired: 1 in, 1 out]
        n157 = call-poly "Enqueue Message.vi"("Priority Message? (F)"=w436, "Message"="Confirm Quit", "Message Queue"=w435) -> ("error out"=w433:errorcluster, "dup Message Queue"=w434:refnum<queue>)  [unwired: 7 in]
        n158 = event-data("Discard?"=TRUE) -> ()  [unwired: 1 in, 1 out]
      }
      event "Exit": Value Change {
        w440 = TRUE  # Priority Message
        # "The UI Message Loop handles sending the Exit message to other loops."
        n159 = event-data() -> ()  [unwired: 1 in, 1 out]
        n160 = call-poly "Enqueue Message.vi"("Priority Message? (F)"=w440, "Message"="Exit", "Message Queue"=w439) -> ("error out"=w444:errorcluster, "dup Message Queue"=w442:refnum<queue>)  [unwired: 7 in]
      }
      event User Event {
        # "The Message Handling Loop processed an \"Exit\" message, which fired this event to stop the Event Handling Loop."
        n161 = event-data() -> ()  [unwired: 1 in, 1 out]
        n162 = local write "Status"("Exit" ("Exit String")) -> ()
      }
      event "Settings Button": Mouse Down {
        # "Allow debugging during run with a ctrl click"
        n163 = event-data() -> ("PlatMods"=w449:T13)  [unwired: 1 in]
        n164 = Unbundle By Name(w449) -> ("Ctrl"=w448:bool)
        n165 = case shown="False" w448 {
          tunnel: [w456 w457] -> w452
          tunnel: [w455 w458] -> w451
          tunnel: w450 -> [w454 w458]
          frame False {
            n166 = call-poly "Enqueue Message.vi"("Message"="Launch Settings Dialog", "Message Queue"=w454) -> ("error out"=w456:errorcluster, "dup Message Queue"=w455:refnum<queue>)  [unwired: 8 in]
          }
          frame True {
            n167 = property class="VI"("BDWin.Open"=TRUE ("Block Diagram Window:Open")) -> (error out=w457:errorcluster)  [unwired: 2 in, 1 out]
          }
        }
      }
      event Key Down {
        n168 = event-data() -> ("ScanCode"=→"ScanCode":i16)  [unwired: 1 in]
      }
    }
    n169 = call "Error Handler - Event Handling Loop.vi"("error in (no error)"=w421, "Message Queue"=w422) -> ("dup error in"=w420:errorcluster)  [unwired: 8 in, 1 out]
  }
  n170 = call "Main Loop.vi"("error in (no error)"=w2, "Chart Notifier"=w17, "Message Queues"=w1) -> ("error out"=w18:errorcluster)  [unwired: 8 in]
  n171 = Unregister For Events(event registration refnum=w25, error in=w30) -> (error out=w26:errorcluster)
  n172 = Close Reference(reference=w16) -> ()  [unwired: 1 in, 1 out]
  n173 = Merge Errors(w26, w31, w2, w18) -> (w29:errorcluster)
  n174 = call "Destroy User Event - Stop.vi"("error in (no error)"=w29, "User Event - Stop"=w27) -> ("error out"=w6:errorcluster)  [unwired: 9 in]
  n175 = flat-sequence {
    tunnel: w6 -> [_]
    frame #0 {
      n176 = invoke class="VI" method="FP.Close"() -> ()  [unwired: 3 in, 3 out]
    }
  }
